vi "Get All VS Frame Changes.vi"(8 "error in (no error)":errorcluster, 9 "New Cluster":refnum<k21>, 10 "VS Filtered Change List":T1 {"Incoming"."Missing"."Node Ref" format="%.0x"; "Incoming"."Changed"."Old"."Node Ref" format="%.0x"; "Outgoing"."Missing"."Node Ref" format="%.0x"; "Outgoing"."Changed"."Old"."Node Ref" format="%.0x"}, 11 "TreeControl in":refnum<vi>) -> (0 "error out":errorcluster, 2 "Change":T10 {"Outgoing"."Frames to Update"."Node Ref" format="%.0x"; "Outgoing"."Frames to Delete" format="%.0x"; "Incoming"."Frames to Update"."Node Ref" format="%.0x"; "Incoming"."Frames to Delete" format="%.0x"}, 3 "TreeControl out":refnum<vi>)   [LabVIEW 2025, in "Protection and Counter Addon System Explorer.lvlib"]
uses:
  Protection and Counter Addon System Explorer.lvlib
  Types/CAN Update Results.ctl
  Types/VS Update List.ctl
  <vilib>/NI VeriStand/Custom Device API/Custom Device Item Ref.ctl
  Types/Base Frame Info_NoVS.ctl
  Types/Signal Attributes.ctl
  Types/CAN Filter Type.ctl
  Types/CAN Frame Update Results.ctl
  Types/Filtered XNET Changes.ctl
  Types/Database Changes.ctl
  Types/Base Frame Info.ctl
  Types/Related CAN Frames.ctl
  Types/Related CAN Frames No VS.ctl
  <vilib>/NI VeriStand/Custom Device API/Custom Device API.lvlib
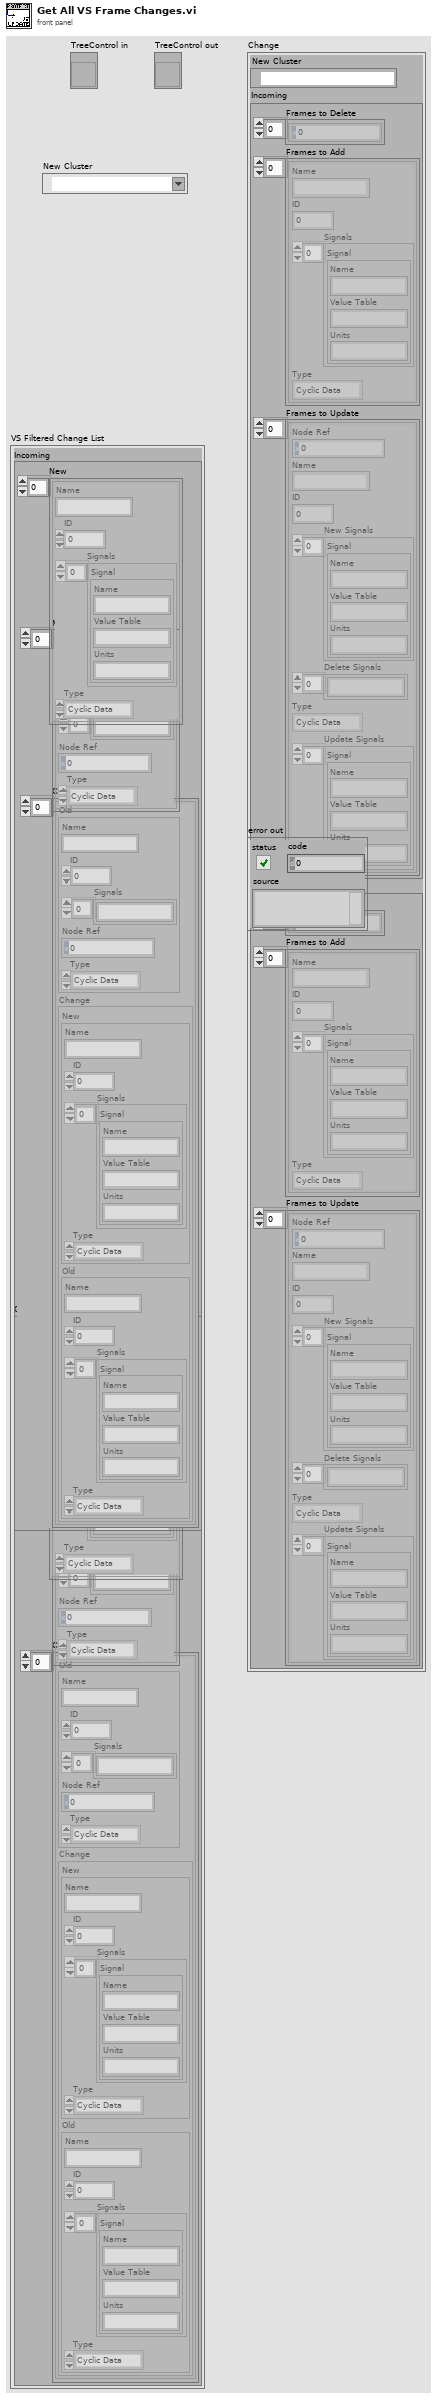
[diagram p1: front panel]
types:
  T1 = typedef "Protection and Counter Addon System Explorer.lvlib/Filtered XNET Changes.ctl" = cluster{"Incoming":T2, "Outgoing":T2}
  T2 = typedef "Protection and Counter Addon System Explorer.lvlib/Database Changes.ctl" = cluster{"New":T3[], "Missing":T6[], "Changed":T8[]}
  T3 = typedef "Protection and Counter Addon System Explorer.lvlib/Base Frame Info_NoVS.ctl" = cluster{"Name":string, "ID":u32, "Signals":T4[], "Type":T5}
  T4 = typedef "Protection and Counter Addon System Explorer.lvlib/Signal Attributes.ctl" = cluster{"Name":string, "Value Table":string, "Units":string}
  T5 = typedef "Protection and Counter Addon System Explorer.lvlib/CAN Filter Type.ctl" = enum16{"Cyclic Data", "Event Data", "Cyclic/Event", "All"}
  T6 = typedef "Protection and Counter Addon System Explorer.lvlib/Base Frame Info.ctl" = cluster{"Name":string, "ID":u32, "Signals":string[], "Node Ref":T7, "Type":T5}
  T7 = typedef "Custom Device API.lvlib/Custom Device Item Ref.ctl" = u64
  T8 = typedef "Protection and Counter Addon System Explorer.lvlib/Related CAN Frames.ctl" = cluster{"Old":T6, "Change":T9}
  T9 = typedef "Protection and Counter Addon System Explorer.lvlib/Related CAN Frames No VS.ctl" = cluster{"New":T3, "Old":T3}
  T10 = typedef "Protection and Counter Addon System Explorer.lvlib/CAN Update Results.ctl" = cluster{"New Cluster":refnum<k21>, "Incoming":T11, "Outgoing":T11}
  T11 = typedef "Protection and Counter Addon System Explorer.lvlib/VS Update List.ctl" = cluster{"Frames to Delete":T7[], "Frames to Add":T3[], "Frames to Update":T12[]}
  T12 = typedef "Protection and Counter Addon System Explorer.lvlib/CAN Frame Update Results.ctl" = cluster{"Node Ref":T7, "Name":string, "ID":u32, "New Signals":T4[], "Delete Signals":string[], "Type":T5, "Update Signals":T4[]}
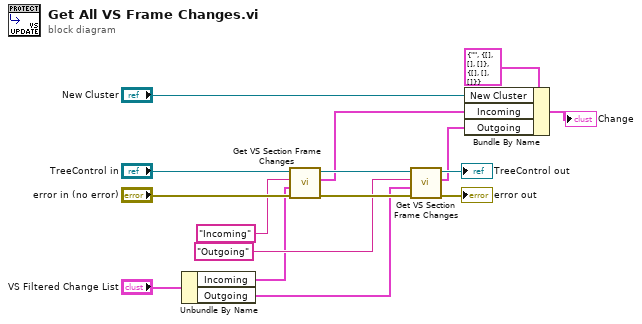
[diagram p0: block diagram]
diagram:
  n1 = Unbundle By Name("VS Filtered Change List") -> ("Incoming"=w5:T2, "Outgoing"=w4:T2)
  n2 = call "Get VS Section Frame Changes.vi"("error in (no error)"="error in (no error)", "Database Changes"=w5, "Section"="Incoming", "TreeControl in"="TreeControl in") -> ("error out"=w11:errorcluster, "Incoming"=w2:T11, "TreeControl out"=w9:refnum<vi>)  [unwired: 5 in]
  n3 = call "Get VS Section Frame Changes.vi"("error in (no error)"=w11, "Database Changes"=w4, "Section"="Outgoing", "TreeControl in"=w9) -> ("error out"=→"error out":errorcluster, "Incoming"=w6:T11, "TreeControl out"=→"TreeControl out":refnum<vi>)  [unwired: 5 in]
  n4 = Bundle By Name(cluster=T10 {"New Cluster"="", "Incoming"={"Frames to Delete"=[], "Frames to Add"=[], "Frames to Update"=[]}, "Outgoing"={"Frames to Delete"=[], "Frames to Add"=[], "Frames to Update"=[]}}, "New Cluster"="New Cluster", "Incoming"=w2, "Outgoing"=w6) -> (→"Change":T10)
